vi "AllocateMemory_u32.vi"(8 "Error In":errorcluster, 9 "Dimension":T1={"Depth"=1, "Height"=1, "Width"=1} {"Width" min=1; "Height" min=1; "Depth" min=1}, 11 "Device In":T3) -> (0 "Error Out":errorcluster, 1 "Dimension Out":T1={"Depth"=1, "Height"=1, "Width"=1} {"Width" min=1; "Height" min=1; "Depth" min=1}, 3 "Memory Object":T2={"Device ID"=0, "Memeroy ID"=0, "Dimension"={"Depth"=1, "Height"=1, "Width"=1}, "Memory Type"=enum."32f"} {"Dimension"."Width" min=1; "Dimension"."Height" min=1; "Dimension"."Depth" min=1})   [LabVIEW 2012, in "OpenCLV x64.lvlib"]
doc: "A VI that allocates u32 memory on the device based on the size of the dimenions. This VI does <b>NOT</b> copy data to the device. Recommended to allocate all memory on the device at the start of the program to avoid device memory fragmentation."
uses:
  OpenCLV x64.lvlib
  Controls/Device ID.ctl
  User Controls/Array Dimensions.ctl
  Controls/Memory Object.ctl
  Controls/Memory ID.ctl
  Controls/Memory Type.ctl
  Error Checking/Add Error Functional Global.vi
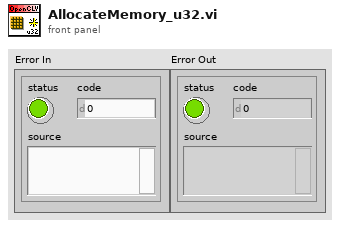
[diagram p1: front panel]
types:
  T1 = typedef "Array Dimensions.ctl" = cluster{"Depth":u64, "Height":u64, "Width":u64}
  T2 = typedef "OpenCLV x64.lvlib/Memory Object.ctl" = cluster{"Device ID":T3, "Memeroy ID":T4, "Dimension":T1, "Memory Type":T5}
  T3 = typedef "OpenCLV x64.lvlib/Device ID.ctl" = u64
  T4 = typedef "OpenCLV x64.lvlib/Memory ID.ctl" = u64
  T5 = typedef "OpenCLV x64.lvlib/Memory Type.ctl" = enum16{"32f", "u8", "i8", "u16", "i16", "u32", "i32", "64f"}
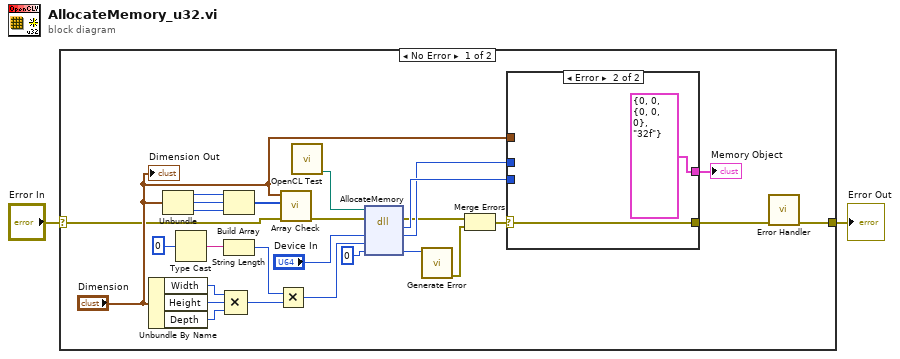
[diagram p0: block diagram]
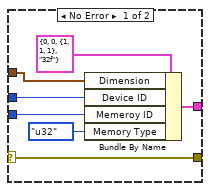
[diagram p2: hidden frame]
diagram:
  n1 = case shown="No Error" "Error In" {
    selector: "Error In" -> [w3 w39]
    tunnel: [w4 w39] -> w1
    frame No Error {
      n2 = Unbundle By Name("Dimension") -> ("Width"=w25:u64, "Height"=w23:u64, "Depth"=w24:u64)
      n3 = Unbundle("Dimension") -> ("Depth"=w8:u64, "Height"=w12:u64, "Width"=w11:u64)
      n4 = Type Cast(x=u32 0) -> (*(type *) &x=w20:string)  [unwired: 1 in]
      n5 = Build Array(w8, w12, w11) -> (w9:u64[])
      n6 = String Length(string=w20) -> (length=w19:i32)
      n7 = Compound Arithmetic op=MULTIPLY(w25, w23, w24) -> (w18:u64)
      n8 = Multiply(x=w19, y=w18) -> (x*y=w17:u64)
      n9 = call "Array Check.vi"("Error In"=w3, "Array Dimensions"=w9, "Vector Dimensions"="Dimension") -> ("error out"=w16:errorcluster)  [unwired: 7 in, 1 out]
      n10 = call "OpenCL Test.vi"() -> ("DLL To Use"=w7:path)  [unwired: 11 in]
      n11 = dll-call lib="C:/Users/bme-amcelroy-la/Desktop/OpenCLV/trunk/OpenCLV_x64_1.0/OpenCLV_x64.dll" fn="AllocateMemory"(path in=w7, error in=w16, "clLabviewDevice"="Device In", "Size Of Data"=w17, "Error"=0) -> (error out=w13:errorcluster, "cl_mem Pointer"=w27:u64, "clLabviewDevice"=w22:u64, "Error"=w26:i32)  [unwired: 2 in, 1 out]
      n12 = call "Generate Error.vi"("Error"=w26) -> ("error out"=w14:errorcluster)  [unwired: 10 in]
      n13 = Merge Errors(w13, w14) -> (w15:errorcluster)
      n14 = case shown="Error" w15 {
        selector: w15 -> [w31 w38]
        tunnel: [w31 w38] -> w5
        tunnel: w27 -> [w32 _]
        tunnel: w22 -> [w35 _]
        tunnel: "Dimension" -> [w34 _]
        tunnel: [w30 T2 {"Device ID"=0, "Memeroy ID"=0, "Dimension"={"Depth"=0, "Height"=0, "Width"=0}, "Memory Type"=enum."32f"} ("Cluster")] -> w6
        frame No Error {
          n15 = Bundle By Name(cluster=T2 {"Device ID"=0, "Memeroy ID"=0, "Dimension"={"Depth"=1, "Height"=1, "Width"=1}, "Memory Type"=enum."32f"} ("Cluster"), "Dimension"=w34, "Device ID"=w35, "Memeroy ID"=w32, "Memory Type"=Memory_Type."u32") -> (w30:T2)
        }
        frame Error {
        }
      }
      "Memory Object" <- w6
      n16 = call-poly "Error Handler.vi"("Error In"=w5) -> ("Error Out"=w4:errorcluster)  [unwired: 10 in]
      "Dimension Out" <- "Dimension"
    }
    frame Error {
    }
  }
  "Error Out" <- w1
